vi "Read Data.vi"(8 "error in (no error)":errorcluster, 11 "Serial Device in":refnum<class "Serial Device.lvclass">) -> (0 "error out":errorcluster, 2 "Channel Data":string[](array[string]), 3 "Serial Device out":refnum<class "Serial Device.lvclass">)   [LabVIEW 2021, in "Serial Hardware.lvlib" / "Serial Device.lvclass"]
uses:
  Serial Device.lvclass
  Serial Device.lvclass/Serial Device.ctl
  Serial Hardware.lvlib
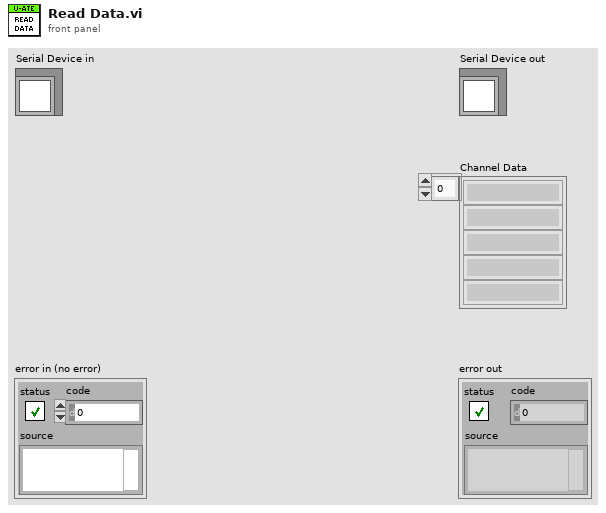
[diagram p1: front panel]
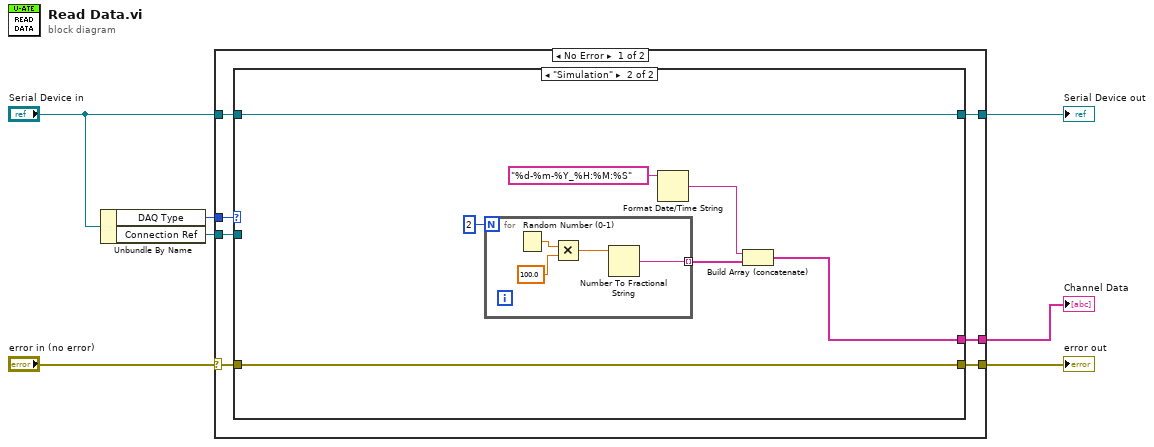
[diagram p0: block diagram]
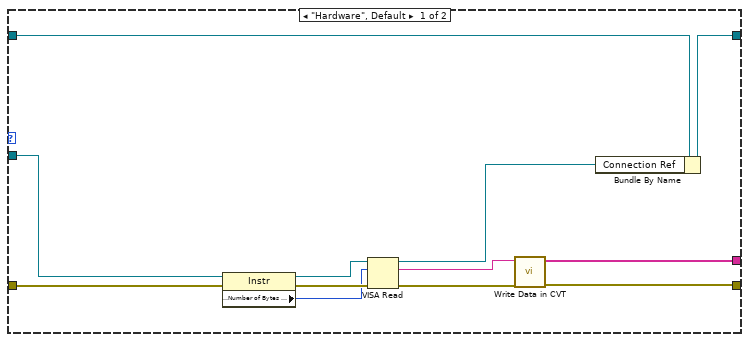
[diagram p2: hidden frame]
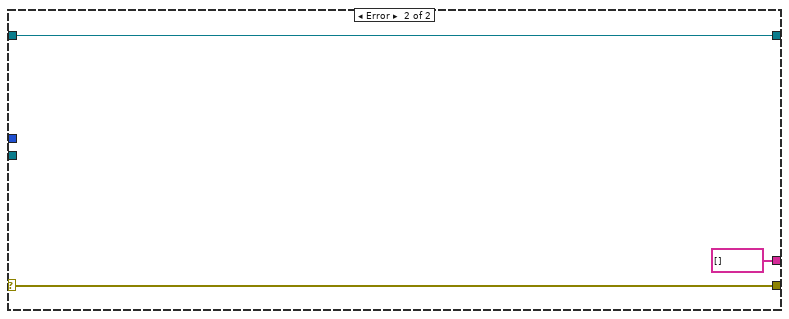
[diagram p3: hidden frame]
diagram:
  n1 = Unbundle By Name("Serial Device in") -> ("DAQ Type"=w5:enum16{"Hardware", "Simulation"}, "Connection Ref"=w2:refnum<visa-resource-name>)
  n2 = case shown="No Error" "error in (no error)" {
    selector: "error in (no error)" -> [w11 w39]
    tunnel: "Serial Device in" -> [w13 w40]
    tunnel: w5 -> [w14 _]
    tunnel: [w12 w40] -> w4
    tunnel: [w10 w39] -> w3
    tunnel: w2 -> [w9 _]
    tunnel: [w8 string[] [] ("Channel Data")] -> w1
    frame No Error {
      n3 = case shown="\"Simulation\"" w14 {
        tunnel: w13 -> [w26 w33]
        tunnel: [w20 w33] -> w12
        tunnel: w11 -> [w25 w32]
        tunnel: [w16 w32] -> w10
        tunnel: w9 -> [w24 _]
        tunnel: [w15 w29] -> w8
        frame "Hardware", Default {
          n4 = property class="Instr"(reference=w24, error in=w25) -> (reference out=w22:refnum<visa-resource-name>, error out=w23:errorcluster, "Serial Settings:Number of Bytes at Serial Port"=w21:u32)
          n5 = VISA Read(VISA resource name=w22, byte count=w21, error in (no error)=w23) -> (VISA resource name out=w19:refnum<visa-resource-name>, read buffer=w17:string, error out=w18:errorcluster)  [unwired: 1 out]
          n6 = call "Write Data in CVT.vi"("error in (no error)"=w18, "Read Buffer"=w17) -> ("error out"=w16:errorcluster, "Channel Data"=w15:string[])  [unwired: 8 in]
          n7 = Bundle By Name(cluster=w26, "Connection Ref"=w19) -> (w20:refnum<class "Serial Device.lvclass">)
        }
        frame "Simulation" {
          n8 = for {
            N: 2 -> [_]
            tunnel: [w34] -> w30 mode=indexing
            n9 = Random Number (0-1)() -> (number: 0 to 1=w37:dbl)
            n10 = Multiply(x=w37, y=100.0) -> (x*y=w35:dbl)
            n11 = Number To Fractional String(number=w35) -> (F-format string=w34:string)  [unwired: 3 in]
          }
          n12 = Format Date/Time String(time format string (%c)="%d-%m-%Y_%H:%M:%S") -> (date/time string=w28:string)  [unwired: 2 in]
          n13 = Build Array (concatenate)(w28, w30) -> (w29:string[])
        }
      }
    }
    frame Error {
    }
  }
  "error out" <- w3
  "Serial Device out" <- w4
  "Channel Data" <- w1
